vi "FuncImg-ROI strings & type.vi"(9 "ROI number":i32, 11 "ROI visibility cluster":T2 {"ROI number" min=1 format="ROI %.0f"}) -> (1 "Plot name":string, 2 "ROI type":T1, 3 "ROI ID string":string)   [LabVIEW 2013]
uses:
  xcontrol/Interface VIs/Interface typedefs/Interface-ROI selection cluster.ctl
  Typedefs/ROI ID Enum.ctl
  xcontrol/Interface VIs/Interface typedefs/Interface-ROI type enum.ctl
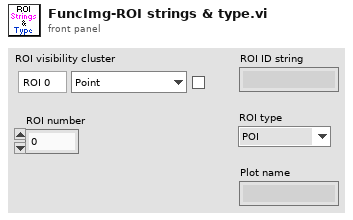
[diagram p1: front panel]
types:
  T1 = typedef "Interface-ROI type enum.ctl" = enum16{"POI", "Mini-scan"}
  T2 = typedef "Interface-ROI selection cluster.ctl" = cluster{"ROI number":i32, "ROI ID":T3, "Visibility":bool}
  T3 = typedef "ROI ID Enum.ctl" = enum16{"Point", "MiniScan", "Comp. MiniScan", "Rectangle", "Comp. volume", "Arb. plane point"}
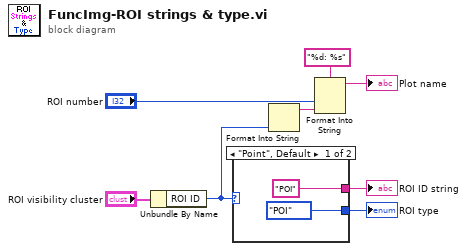
[diagram p0: block diagram]
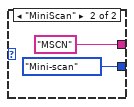
[diagram p2: hidden frame]
diagram:
  n1 = Unbundle By Name("ROI visibility cluster") -> ("ROI ID"=w6:T3)
  n2 = case shown="\"Point\", Default" w6 {
    tunnel: ["POI" ("input 1") "MSCN" ("input 1")] -> w2
    tunnel: [Interface-ROI_type_enum."POI" ("Type") Interface-ROI_type_enum."Mini-scan" ("Type")] -> w3
    frame "Point", Default {
    }
    frame "MiniScan" {
    }
  }
  "ROI type" <- w3
  "ROI ID string" <- w2
  n3 = Format Into String(w6) -> (resulting string=w8:string)  [unwired: 3 in, 1 out]
  n4 = Format Into String(format string="%d: %s", "ROI number", w8) -> (resulting string=→"Plot name":string)  [unwired: 2 in, 1 out]
